vi "alg_solveLin (SubVI).vi"(8 "에러 입력(에러 없음)":errorcluster, 10 "vector":dbl[](array[numeric]), 11 "matrix":dbl[][](array[numeric])) -> (0 "에러 출력":errorcluster, 2 "ans":dbl[](array[numeric]), 3 "참조 번호 출력":refnum<k35>)   [LabVIEW 2018]
uses:
  PythonConfigGlobal.vi
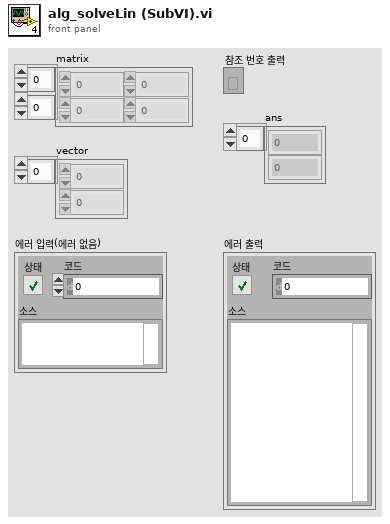
[diagram p1: front panel]
types:
  T1 = cluster{"session out":refnum<k35>, "appended path":path}
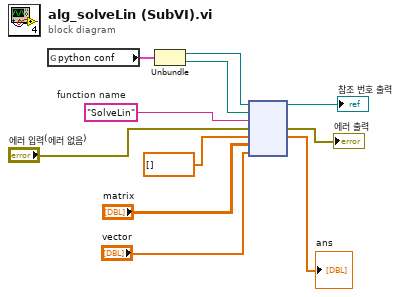
[diagram p0: block diagram]
diagram:
  w7 = "SolveLin"  # function name
  n1 = global read "PythonConfigGlobal.vi" "python conf"() -> (w4:T1)
  n2 = Unbundle(w4) -> ("session out"=w6:refnum<k35>, "appended path"=w5:path)
  n3 = node(w6, w5, w7, "에러 입력(에러 없음)", dbl[] [] ("vector"), "matrix", "vector") -> (→"참조 번호 출력":refnum<k35>, →"에러 출력":errorcluster, →"ans":dbl[])  [unwired: 2 in, 2 out]
